vi "hextofloat.vi"(0 "object in":refnum<class "interface.lvclass">, 1 "数组":u16[](array[numeric]) format="%04xH", 5 "error in (no error)":errorcluster) -> (14 "object out":refnum<class "interface.lvclass">, 15 "FLOAT":sgl[](array[numeric]), 19 "error out":errorcluster)   [LabVIEW 2016, in "interface.lvclass"]
uses:
  interface.lvclass
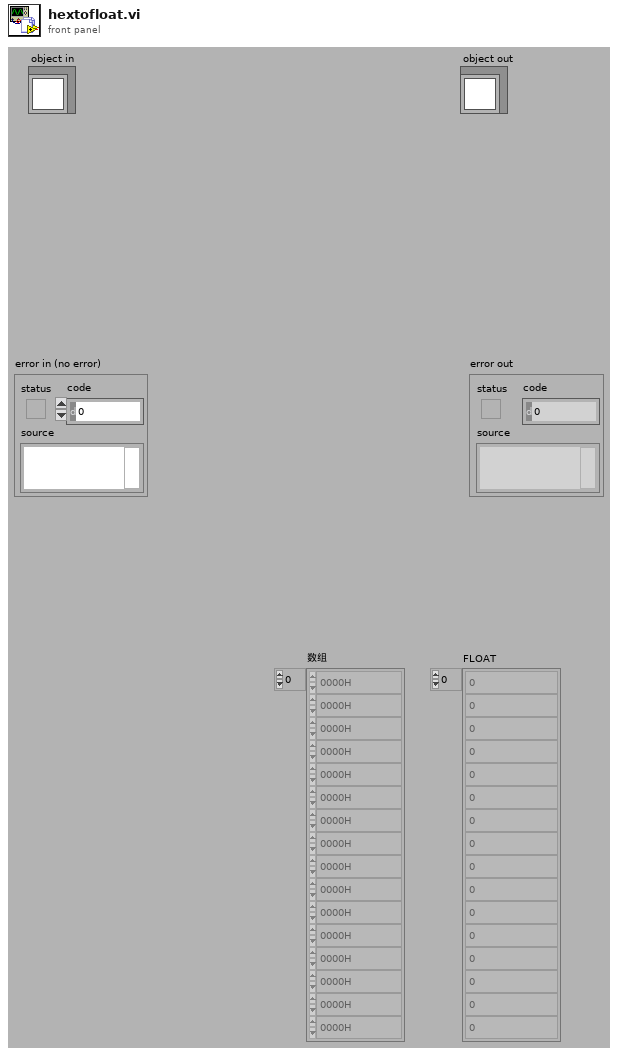
[diagram p1: front panel]
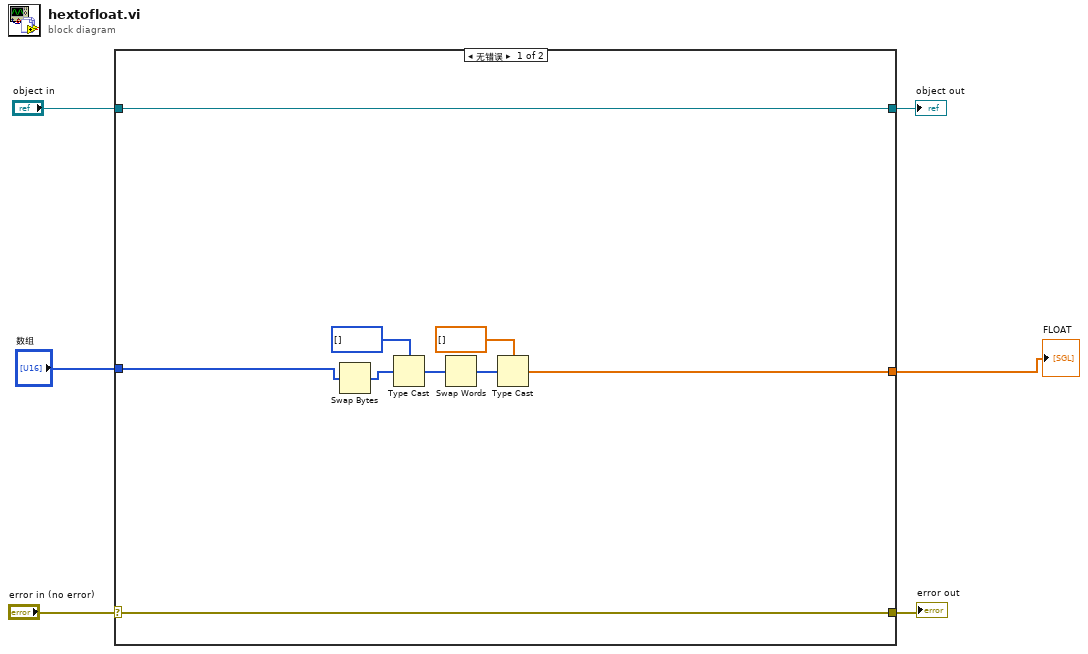
[diagram p0: block diagram]
diagram:
  n1 = case shown="无错误" "error in (no error)" {
    selector: "error in (no error)" -> [w15 w17]
    tunnel: [w15 w17] -> w5
    tunnel: [w14 w16] -> w3
    tunnel: "object in" -> [w14 w16]
    tunnel: "数组" -> [w8 _]
    tunnel: [w7 _] -> w1
    frame No Error {
      n2 = Swap Bytes(anything=w8) -> (byte swapped=w9:u16[])
      n3 = Type Cast(type=u32[] [], x=w9) -> (*(type *) &x=w11:u32[])
      n4 = Swap Words(1:w11) -> (0:w10:u32[])
      n5 = Type Cast(type=sgl[] [], x=w10) -> (*(type *) &x=w7:sgl[])
    }
    frame Error {
    }
  }
  "error out" <- w5
  "object out" <- w3
  "FLOAT" <- w1
